vi "SSC Digital PPMU Measure.vi"(0 "Digital SSC in":T2[](array[typedef]), 5 "Measurement Type":T1=2400 items=["Voltage"=2401, "Current"=2400], 11 "error in":errorcluster) -> (4 "Digital SSC out":T2[](array[typedef]), 6 "Per-Instrument Measurements":dbl[][](array[numeric]), 15 "error out":errorcluster)   [LabVIEW 2019]
doc: "Instructs the PPMU to measure voltage or current on the specified pin(s) and pin group(s). This VI can be called to take a voltage measurement even if the pin function is not set to PPMU."
uses:
  SSC Digital.ctl
  <instrlib>/niDigital/niDigital.llb/niDigital Measurement Type.ctl
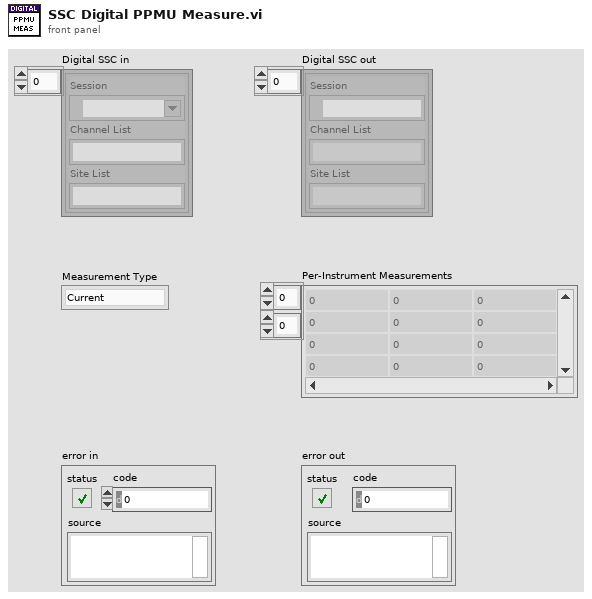
[diagram p1: front panel]
types:
  T1 = typedef "niDigital Measurement Type.ctl" = i32
  T2 = typedef "SSC Digital.ctl" = cluster{"Session":refnum<k15>, "Channel List":string, "Site List":string}
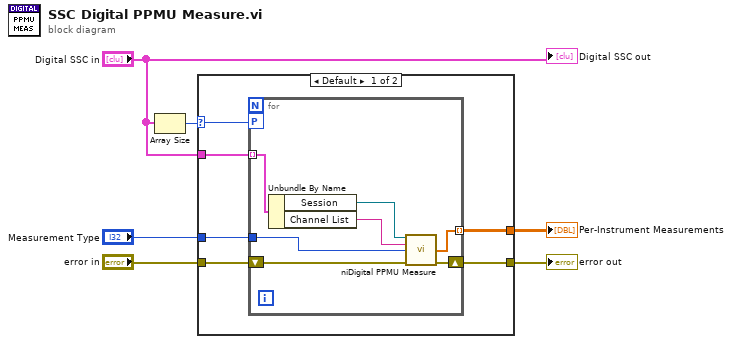
[diagram p0: block diagram]
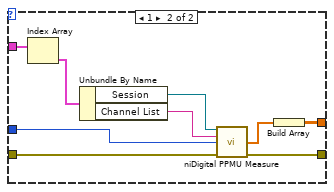
[diagram p2: hidden frame]
diagram:
  n1 = Array Size(array="Digital SSC in") -> (size(s)=w2:i32)
  n2 = case shown="Default" w2 {
    selector: w2 -> [w8 _]
    tunnel: [w12 w20] -> w6
    tunnel: "error in" -> [w11 w27]
    tunnel: [w10 w26] -> w4
    tunnel: "Measurement Type" -> [w9 w25]
    tunnel: "Digital SSC in" -> [w7 w24]
    frame Default {
      n3 = for {
        tunnel: w7 -> [w16] mode=indexing
        tunnel: [w17] -> w12 mode=indexing
        workers-P: w8 -> [_]
        shift-right: [w18] -> w10
        shift-left: w11 -> [w19]
        tunnel: w9 -> [w13]
        n4 = Unbundle By Name(w16) -> ("Session"=w15:refnum<k15>, "Channel List"=w14:string)
        n5 = call <instrlib>:"niDigital PPMU Measure.vi"("instrument handle"=w15, "channel list"=w14, "measurement type"=w13, "error in"=w19) -> ("measurements"=w17:dbl[], "error out"=w18:errorcluster)  [unwired: 9 in, 1 out]
      }
    }
    frame 1 {
      n6 = Index Array(array=w24) -> (element=w21:T2)  [unwired: 1 in]
      n7 = Unbundle By Name(w21) -> ("Session"=w23:refnum<k15>, "Channel List"=w22:string)
      n8 = call <instrlib>:"niDigital PPMU Measure.vi"("instrument handle"=w23, "channel list"=w22, "measurement type"=w25, "error in"=w27) -> ("measurements"=w28:dbl[], "error out"=w26:errorcluster)  [unwired: 9 in, 1 out]
      n9 = Build Array(w28) -> (w20:dbl[][])
    }
  }
  "error out" <- w4
  "Per-Instrument Measurements" <- w6
  "Digital SSC out" <- "Digital SSC in"
